vi "SSC DAQmx Commit.vi"(0 "DAQmx SSC in":T1[](array[typedef]), 11 "error in":errorcluster) -> (4 "DAQmx SSC out":T1[](array[typedef]), 15 "error out":errorcluster)   [LabVIEW 2020]
doc: "Applies previously configured settings to the device. Calling this VI moves the NI-DAQmx tasks from the Uncommitted state into the Committed state."
uses:
  Pin Map/SSC DAQmx.ctl
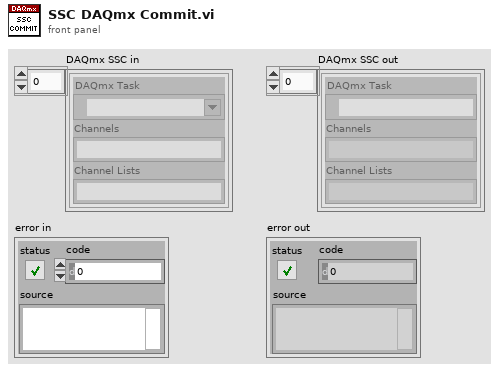
[diagram p1: front panel]
types:
  T1 = typedef "SSC DAQmx.ctl" = cluster{"DAQmx Task ":refnum<k21>, "Channels":string, "Channel Lists":string}
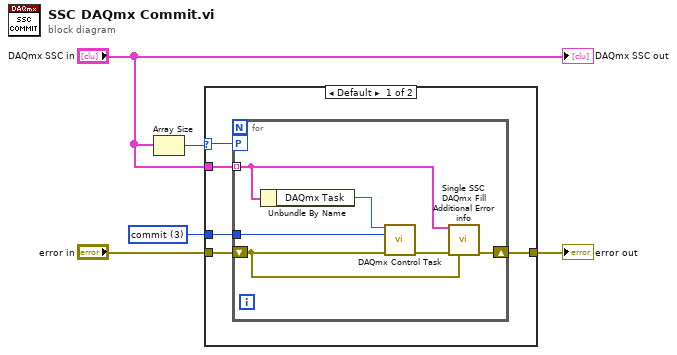
[diagram p0: block diagram]
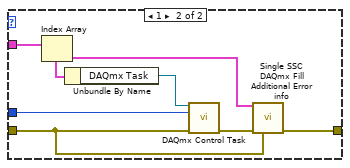
[diagram p2: hidden frame]
diagram:
  w1 = 3 items=["verify"=2, "reserve"=4, "commit"=3, "unreserve"=5, "abort"=6] ("action")
  n1 = Array Size(array="DAQmx SSC in") -> (size(s)=w3:i32)
  n2 = case shown="Default" w3 {
    selector: w3 -> [w8 _]
    tunnel: [w10 w22] -> w5
    tunnel: "error in" -> [w9 w20]
    tunnel: "DAQmx SSC in" -> [w7 w23]
    tunnel: w1 -> [w6 w17]
    frame Default {
      n3 = for {
        tunnel: w7 -> [w13] mode=indexing
        workers-P: w8 -> [_]
        shift-right: [w16] -> w10
        shift-left: w9 -> [w15]
        tunnel: w6 -> [w11]
        n4 = Unbundle By Name(w13) -> ("DAQmx Task"=w12:refnum<k21>)
        n5 = call <vilib>:"DAQmx Control Task.vi"("task/channels in"=w12, "action"=w11, "error in"=w15) -> ("error out"=w14:errorcluster)  [unwired: 11 in, 1 out]
        n6 = call "Single SSC DAQmx Fill Additional Error info.vi"("DAQmx SSC in"=w13, "error in"=w14, "previous error in"=w15) -> ("error out"=w16:errorcluster)  [unwired: 12 in]
      }
    }
    frame 1 {
      n7 = Index Array(array=w23) -> (element=w18:T1)  [unwired: 1 in]
      n8 = Unbundle By Name(w18) -> ("DAQmx Task"=w21:refnum<k21>)
      n9 = call <vilib>:"DAQmx Control Task.vi"("task/channels in"=w21, "action"=w17, "error in"=w20) -> ("error out"=w19:errorcluster)  [unwired: 11 in, 1 out]
      n10 = call "Single SSC DAQmx Fill Additional Error info.vi"("DAQmx SSC in"=w18, "error in"=w19, "previous error in"=w20) -> ("error out"=w22:errorcluster)  [unwired: 12 in]
    }
  }
  "error out" <- w5
  "DAQmx SSC out" <- "DAQmx SSC in"
